vi "Configure Digital Input Noise Power.vi"(6 "Total Noise Power (-2.03030000E+002)":dbl=-203.03 format="%.8e", 7 "Channel Noise Power (-1.44000000E+002 dBm)":dbl=-144.0 format="%.8e", 8 "error in (no error)":errorcluster, 9 "Carrier Power (-1.44000000E+002)":dbl=-144.0 format="%.8e", 10 "Power Control Mode (0: Total)":i32(ring) items=["Total", "Carrier", "Total Noise", "N Channel"], 11 "VISA resource name":refnum<visa-resource-name>) -> (0 "error out":errorcluster, 3 "VISA resource name out":refnum<visa-resource-name>)   [LabVIEW 2018, in "Agilent PSG MXG Series.lvlib"]
doc: "Configures the digital input noise power settings.\n\n<b>Note:</b>\nIt is applicable for N5172B/82B with <b>Option 004</b> only."
uses:
  Agilent PSG MXG Series.lvlib
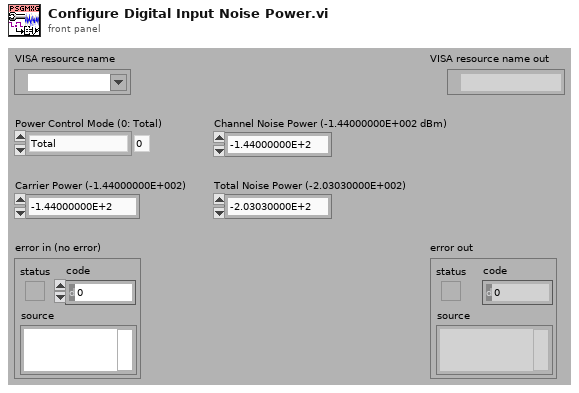
[diagram p1: front panel]
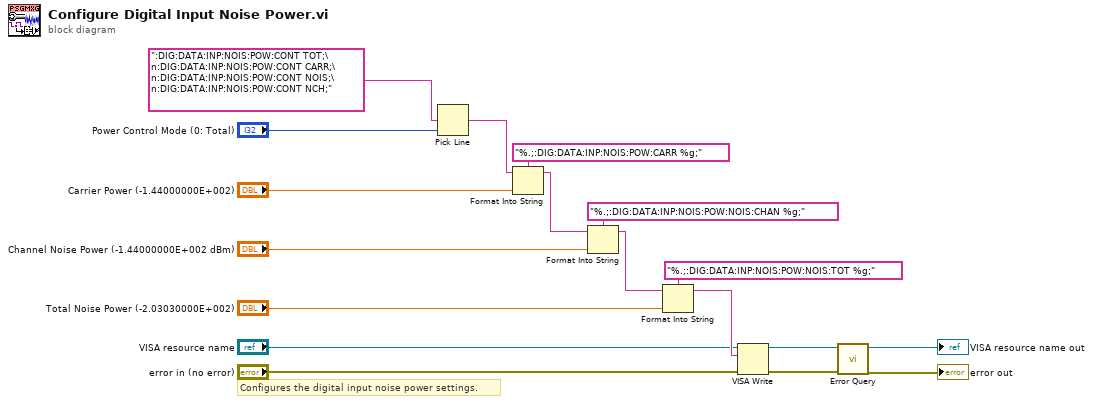
[diagram p0: block diagram]
diagram:
  # "Configures the digital input noise power settings."
  n1 = Pick Line(multi-line string=":DIG:DATA:INP:NOIS:POW:CONT TOT;\n:DIG:DATA:INP:NOIS:POW:CONT CARR;\n:DIG:DATA:INP:NOIS:POW:CONT NOIS;\n:DIG:DATA:INP:NOIS:POW:CONT NCH;", line index="Power Control Mode (0: Total)") -> (output string=w16:string)  [unwired: 1 in]
  n2 = Format Into String(format string="%.;:DIG:DATA:INP:NOIS:POW:CARR %g;", initial string=w16, "Carrier Power (-1.44000000E+002)") -> (resulting string=w13:string)  [unwired: 1 in, 1 out]
  n3 = Format Into String(format string="%.;:DIG:DATA:INP:NOIS:POW:NOIS:CHAN %g;", initial string=w13, "Channel Noise Power (-1.44000000E+002 dBm)") -> (resulting string=w10:string)  [unwired: 1 in, 1 out]
  n4 = Format Into String(format string="%.;:DIG:DATA:INP:NOIS:POW:NOIS:TOT %g;", initial string=w10, "Total Noise Power (-2.03030000E+002)") -> (resulting string=w7:string)  [unwired: 1 in, 1 out]
  n5 = VISA Write(VISA resource name="VISA resource name", write buffer=w7, error in (no error)="error in (no error)") -> (VISA resource name out=w4:refnum<visa-resource-name>, error out=w3:errorcluster)  [unwired: 1 out]
  n6 = call "Error Query.vi"("error in (no error)"=w3, "VISA resource name"=w4) -> ("error out"=→"error out":errorcluster, "VISA resource name out"=→"VISA resource name out":refnum<visa-resource-name>)  [unwired: 6 in, 2 out]
